vi "MergeJSONData.vi"(8 "Telemetry":cluster{"Name":string[], "Value":string[]}, 11 "JSON Telemetry":string) -> (0 "TelemetryOut":cluster{"Name":string[], "Value":string[]})   [LabVIEW 2014]
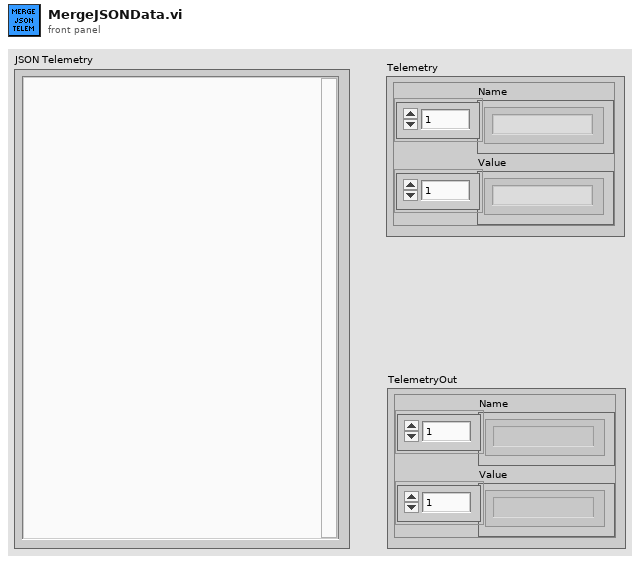
[diagram p1: front panel]
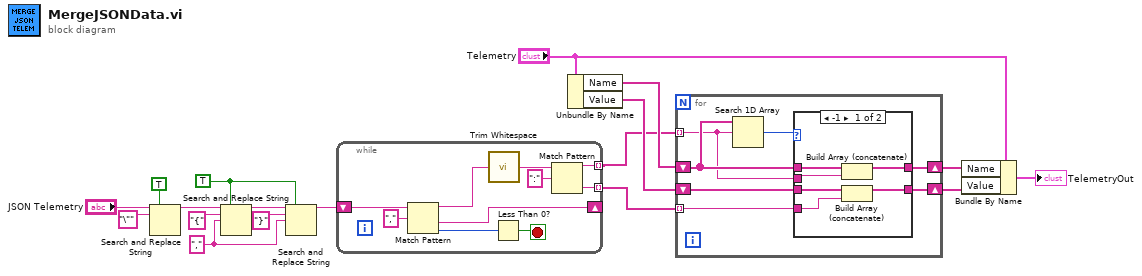
[diagram p0: block diagram]
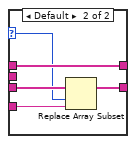
[diagram p2: hidden frame]
diagram:
  w18 = ","
  w15 = TRUE ("replace all? (F)")
  n1 = Search and Replace String(replace all?=TRUE ("replace all? (F)"), input string="JSON Telemetry", search string="\"") -> (result string=w8:string)  [unwired: 5 in, 3 out]
  n2 = Search and Replace String(replace all?=w15, input string=w8, search string="{", replace string=w18) -> (result string=w14:string)  [unwired: 4 in, 3 out]
  n3 = Search and Replace String(replace all?=w15, input string=w14, search string="}", replace string=w18) -> (result string=w13:string)  [unwired: 4 in, 3 out]
  n4 = while {
    shift-right: [w28] -> _
    shift-left: w13 -> [w19]
    tunnel: [w21] -> w2 mode=indexing
    tunnel: [w20] -> w1 mode=indexing
    stop <- w25 stop-if-true
    n5 = Match Pattern(string=w19, regular expression=",") -> (before substring=w27:string, after substring=w28:string, offset past match=w26:i32)  [unwired: 1 in, 1 out]
    n6 = call <vilib>:"Trim Whitespace.vi"("string"=w27) -> ("trimmed string"=w23:string)  [unwired: 1 in]
    n7 = Less Than 0?(x=w26) -> (x < 0?=w25:bool)
    n8 = Match Pattern(string=w23, regular expression=":") -> (before substring=w21:string, after substring=w20:string)  [unwired: 1 in, 2 out]
  }
  n9 = Unbundle By Name("Telemetry") -> ("Name"=w4:string[], "Value"=w3:string[])
  n10 = for {
    tunnel: w2 -> [w29] mode=indexing
    shift-right: [w32] -> w11
    shift-left: w4 -> [w33]
    shift-right: [w30] -> w10
    shift-left: w3 -> [w31]
    tunnel: w1 -> [w34] mode=indexing
    n11 = Search 1D Array(1D array=w33, element=w29) -> (index of element=w35:i32)  [unwired: 1 in]
    n12 = case shown="-1" w35 {
      selector: w35 -> [_ w44]
      tunnel: w34 -> [w37 w43]
      tunnel: [w39 w46] -> w32
      tunnel: w33 -> [w41 w46]
      tunnel: w31 -> [w38 w45]
      tunnel: [w36 w42] -> w30
      tunnel: w29 -> [w40 _]
      frame -1 {
        n13 = Build Array (concatenate)(w41, w40) -> (w39:string[])
        n14 = Build Array (concatenate)(w38, w37) -> (w36:string[])
      }
      frame Default {
        n15 = Replace Array Subset(array=w45, new element=w43, index=w44) -> (w42:string[])
      }
    }
  }
  n16 = Bundle By Name(cluster="Telemetry", "Name"=w11, "Value"=w10) -> (→"TelemetryOut":cluster{"Name":string[], "Value":string[]})
